vi "Configure9219.vi"(7 "Channel Number":i32, 8 "error in (no error)":errorcluster, 9 "ChannelType":string, 10 "Properties":T1[](array[typedef]), 11 "IO Ref in":refnum<k21>) -> (0 "error out":errorcluster, 3 "IO Ref out":refnum<k21>)   [LabVIEW 2017, in "ScanEngine.lvlib"]
uses:
  <vilib>/addons/InsightCM/Devices/Shared/Common/ScanEngine/ScanEngine.lvlib
  <vilib>/addons/InsightCM/MessageBus/Base/controls/KeyValuePair.ctl
  <resource>/objmgr/cRIO.rc
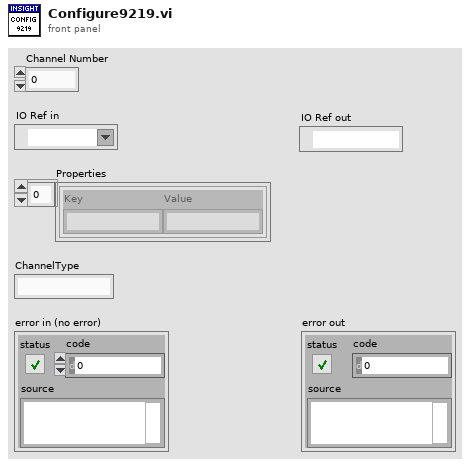
[diagram p1: front panel]
types:
  T1 = typedef "KeyValuePair.ctl" = cluster{"Key":string, "Value":string}
  T2 = cluster{"Degree":u32, "DigThresh":dbl, "RangeMode":u32, "RTD type":u32, "A":dbl, "B":dbl, "C":dbl, "r0":dbl, "TC Type":u32}
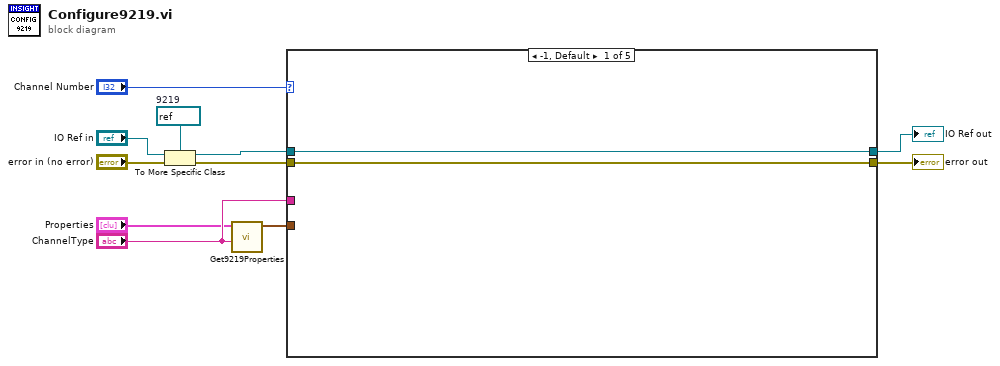
[diagram p0: block diagram]
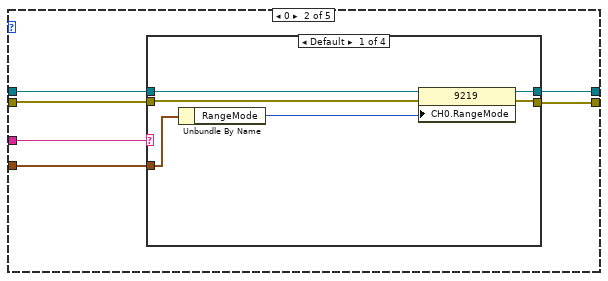
[diagram p2: hidden frame]
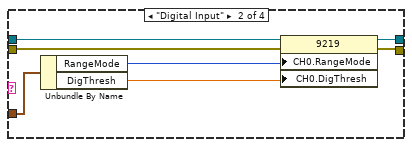
[diagram p3: hidden frame]
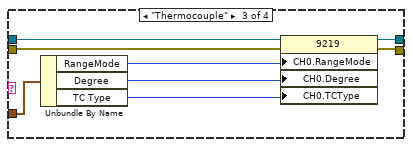
[diagram p4: hidden frame]
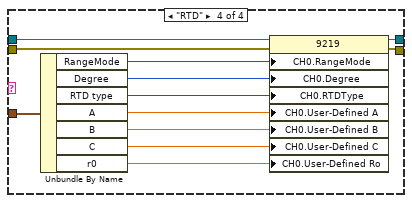
[diagram p5: hidden frame]
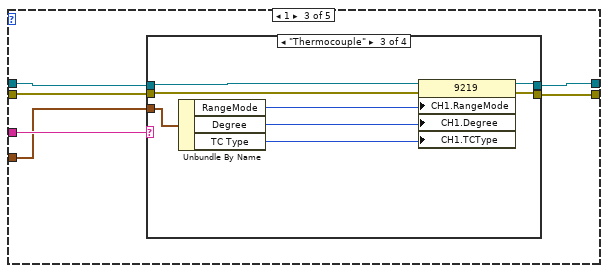
[diagram p6: hidden frame]
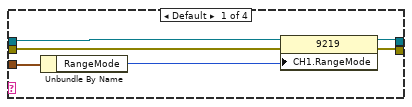
[diagram p7: hidden frame]
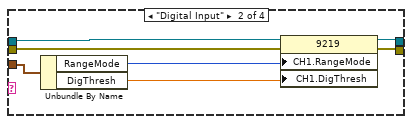
[diagram p8: hidden frame]
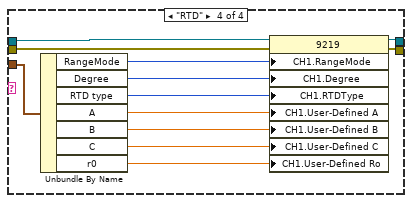
[diagram p9: hidden frame]
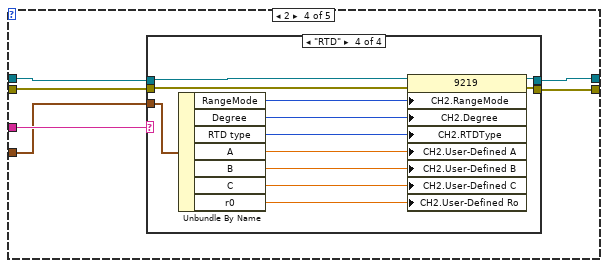
[diagram p10: hidden frame]
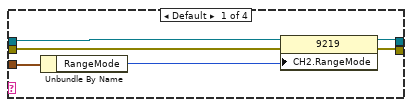
[diagram p11: hidden frame]
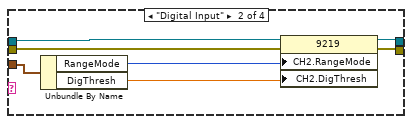
[diagram p12: hidden frame]
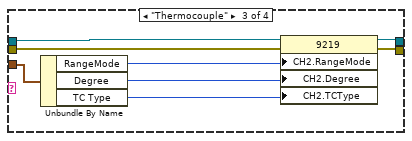
[diagram p13: hidden frame]
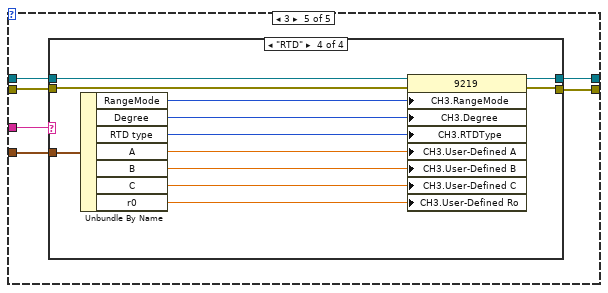
[diagram p14: hidden frame]
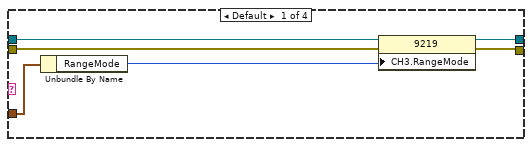
[diagram p15: hidden frame]
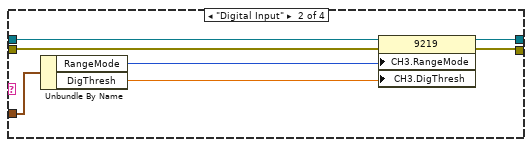
[diagram p16: hidden frame]
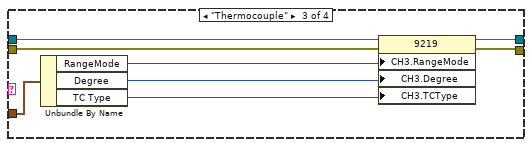
[diagram p17: hidden frame]
diagram:
  w5 = refnum<k21> refnum  # 9219
  n1 = To More Specific Class(target class=w5, reference="IO Ref in", error in="error in (no error)") -> (specific class reference=w4:refnum<k21>, error out=w10:errorcluster)
  n2 = call <vilib>:"Get9219Properties.vi"("ChannelType"="ChannelType", "Properties"="Properties") -> ("9219 Channel Settings"=w9:T2)  [unwired: 9 in]
  n3 = case shown="-1, Default" "Channel Number" {
    tunnel: w10 -> [w13 w16 w55 w94 w133]
    tunnel: [w13 w19 w58 w97 w136] -> w1
    tunnel: w4 -> [w12 w18 w57 w96 w135]
    tunnel: [w12 w17 w56 w95 w134] -> w6
    tunnel: w9 -> [_ w14 w53 w92 w131]
    tunnel: "ChannelType" -> [_ w15 w54 w93 w132]
    frame -1, Default {
    }
    frame 0 {
      n4 = case shown="Default" w15 {
        tunnel: [w23 w30 w38 w50] -> w19
        tunnel: w18 -> [w22 w29 w37 w49]
        tunnel: [w24 w31 w39 w51] -> w17
        tunnel: w16 -> [w21 w28 w36 w48]
        tunnel: w14 -> [w20 w27 w35 w47]
        frame Default {
          n5 = Unbundle By Name(w20) -> ("RangeMode"=w25:u32)
          n6 = property class="9219"(reference=w22, error in=w21, "CH0.RangeMode"=w25) -> (reference out=w24:refnum<k21>, error out=w23:errorcluster)
        }
        frame "Digital Input" {
          n7 = Unbundle By Name(w27) -> ("RangeMode"=w32:u32, "DigThresh"=w26:dbl)
          n8 = property class="9219"(reference=w29, error in=w28, "CH0.RangeMode"=w32, "CH0.DigThresh"=w26) -> (reference out=w31:refnum<k21>, error out=w30:errorcluster)
        }
        frame "Thermocouple" {
          n9 = Unbundle By Name(w35) -> ("RangeMode"=w40:u32, "Degree"=w34:u32, "TC Type"=w33:u32)
          n10 = property class="9219"(reference=w37, error in=w36, "CH0.RangeMode"=w40, "CH0.Degree"=w34, "CH0.TCType"=w33) -> (reference out=w39:refnum<k21>, error out=w38:errorcluster)
        }
        frame "RTD" {
          n11 = Unbundle By Name(w47) -> ("RangeMode"=w52:u32, "Degree"=w46:u32, "RTD type"=w45:u32, "A"=w44:dbl, "B"=w43:dbl, "C"=w42:dbl, "r0"=w41:dbl)
          n12 = property class="9219"(reference=w49, error in=w48, "CH0.RangeMode"=w52, "CH0.Degree"=w46, "CH0.RTDType"=w45, "CH0.User-Defined A"=w44, "CH0.User-Defined B"=w43, "CH0.User-Defined C"=w42, "CH0.User-Defined Ro"=w41) -> (reference out=w51:refnum<k21>, error out=w50:errorcluster)
        }
      }
    }
    frame 1 {
      n13 = case shown="\"Thermocouple\"" w54 {
        tunnel: [w62 w69 w77 w89] -> w58
        tunnel: w57 -> [w61 w68 w76 w88]
        tunnel: [w63 w70 w78 w90] -> w56
        tunnel: w55 -> [w60 w67 w75 w87]
        tunnel: w53 -> [w59 w66 w74 w86]
        frame Default {
          n14 = Unbundle By Name(w59) -> ("RangeMode"=w64:u32)
          n15 = property class="9219"(reference=w61, error in=w60, "CH1.RangeMode"=w64) -> (reference out=w63:refnum<k21>, error out=w62:errorcluster)
        }
        frame "Digital Input" {
          n16 = Unbundle By Name(w66) -> ("RangeMode"=w71:u32, "DigThresh"=w65:dbl)
          n17 = property class="9219"(reference=w68, error in=w67, "CH1.RangeMode"=w71, "CH1.DigThresh"=w65) -> (reference out=w70:refnum<k21>, error out=w69:errorcluster)
        }
        frame "Thermocouple" {
          n18 = Unbundle By Name(w74) -> ("RangeMode"=w79:u32, "Degree"=w73:u32, "TC Type"=w72:u32)
          n19 = property class="9219"(reference=w76, error in=w75, "CH1.RangeMode"=w79, "CH1.Degree"=w73, "CH1.TCType"=w72) -> (reference out=w78:refnum<k21>, error out=w77:errorcluster)
        }
        frame "RTD" {
          n20 = Unbundle By Name(w86) -> ("RangeMode"=w91:u32, "Degree"=w85:u32, "RTD type"=w84:u32, "A"=w83:dbl, "B"=w82:dbl, "C"=w81:dbl, "r0"=w80:dbl)
          n21 = property class="9219"(reference=w88, error in=w87, "CH1.RangeMode"=w91, "CH1.Degree"=w85, "CH1.RTDType"=w84, "CH1.User-Defined A"=w83, "CH1.User-Defined B"=w82, "CH1.User-Defined C"=w81, "CH1.User-Defined Ro"=w80) -> (reference out=w90:refnum<k21>, error out=w89:errorcluster)
        }
      }
    }
    frame 2 {
      n22 = case shown="\"RTD\"" w93 {
        tunnel: [w101 w108 w116 w128] -> w97
        tunnel: w96 -> [w100 w107 w115 w127]
        tunnel: [w102 w109 w117 w129] -> w95
        tunnel: w94 -> [w99 w106 w114 w126]
        tunnel: w92 -> [w98 w105 w113 w125]
        frame Default {
          n23 = Unbundle By Name(w98) -> ("RangeMode"=w103:u32)
          n24 = property class="9219"(reference=w100, error in=w99, "CH2.RangeMode"=w103) -> (reference out=w102:refnum<k21>, error out=w101:errorcluster)
        }
        frame "Digital Input" {
          n25 = Unbundle By Name(w105) -> ("RangeMode"=w110:u32, "DigThresh"=w104:dbl)
          n26 = property class="9219"(reference=w107, error in=w106, "CH2.RangeMode"=w110, "CH2.DigThresh"=w104) -> (reference out=w109:refnum<k21>, error out=w108:errorcluster)
        }
        frame "Thermocouple" {
          n27 = Unbundle By Name(w113) -> ("RangeMode"=w118:u32, "Degree"=w112:u32, "TC Type"=w111:u32)
          n28 = property class="9219"(reference=w115, error in=w114, "CH2.RangeMode"=w118, "CH2.Degree"=w112, "CH2.TCType"=w111) -> (reference out=w117:refnum<k21>, error out=w116:errorcluster)
        }
        frame "RTD" {
          n29 = Unbundle By Name(w125) -> ("RangeMode"=w130:u32, "Degree"=w124:u32, "RTD type"=w123:u32, "A"=w122:dbl, "B"=w121:dbl, "C"=w120:dbl, "r0"=w119:dbl)
          n30 = property class="9219"(reference=w127, error in=w126, "CH2.RangeMode"=w130, "CH2.Degree"=w124, "CH2.RTDType"=w123, "CH2.User-Defined A"=w122, "CH2.User-Defined B"=w121, "CH2.User-Defined C"=w120, "CH2.User-Defined Ro"=w119) -> (reference out=w129:refnum<k21>, error out=w128:errorcluster)
        }
      }
    }
    frame 3 {
      n31 = case shown="\"RTD\"" w132 {
        tunnel: [w140 w147 w155 w168] -> w136
        tunnel: w135 -> [w139 w146 w154 w167]
        tunnel: [w141 w148 w156 w169] -> w134
        tunnel: w133 -> [w138 w145 w153 w166]
        tunnel: w131 -> [w137 w144 w152 w165]
        frame Default {
          n32 = Unbundle By Name(w137) -> ("RangeMode"=w142:u32)
          n33 = property class="9219"(reference=w139, error in=w138, "CH3.RangeMode"=w142) -> (reference out=w141:refnum<k21>, error out=w140:errorcluster)
        }
        frame "Digital Input" {
          n34 = Unbundle By Name(w144) -> ("RangeMode"=w149:u32, "DigThresh"=w143:dbl)
          n35 = property class="9219"(reference=w146, error in=w145, "CH3.RangeMode"=w149, "CH3.DigThresh"=w143) -> (reference out=w148:refnum<k21>, error out=w147:errorcluster)
        }
        frame "Thermocouple" {
          n36 = Unbundle By Name(w152) -> ("RangeMode"=w157:u32, "Degree"=w151:u32, "TC Type"=w150:u32)
          n37 = property class="9219"(reference=w154, error in=w153, "CH3.RangeMode"=w157, "CH3.Degree"=w151, "CH3.TCType"=w150) -> (reference out=w156:refnum<k21>, error out=w155:errorcluster)
        }
        frame "RTD" {
          n38 = Unbundle By Name(w165) -> ("RangeMode"=w164:u32, "Degree"=w163:u32, "RTD type"=w162:u32, "A"=w161:dbl, "B"=w160:dbl, "C"=w159:dbl, "r0"=w158:dbl)
          n39 = property class="9219"(reference=w167, error in=w166, "CH3.RangeMode"=w164, "CH3.Degree"=w163, "CH3.RTDType"=w162, "CH3.User-Defined A"=w161, "CH3.User-Defined B"=w160, "CH3.User-Defined C"=w159, "CH3.User-Defined Ro"=w158) -> (reference out=w169:refnum<k21>, error out=w168:errorcluster)
        }
      }
    }
  }
  "IO Ref out" <- w6
  "error out" <- w1
